vi "LFA_Close.vi"(8 "error in (no error)":errorcluster, 11 "LightField Automation in":refnum<class "LightField Automation.lvclass">) -> (0 "error out":errorcluster, 3 "LightField Automation out":refnum<class "LightField Automation.lvclass">)   [LabVIEW 2013, in "LightField Automation.lvclass"]
uses:
  LightField Automation.lvclass
  LightField Automation.lvclass/LightField Automation.ctl
  C:/Program Files/Princeton Instruments/LightField/PrincetonInstruments.LightField.AutomationV3.dll
  Program Files/Princeton Instruments/LightField/PrincetonInstruments.LightField.AutomationV3.dll
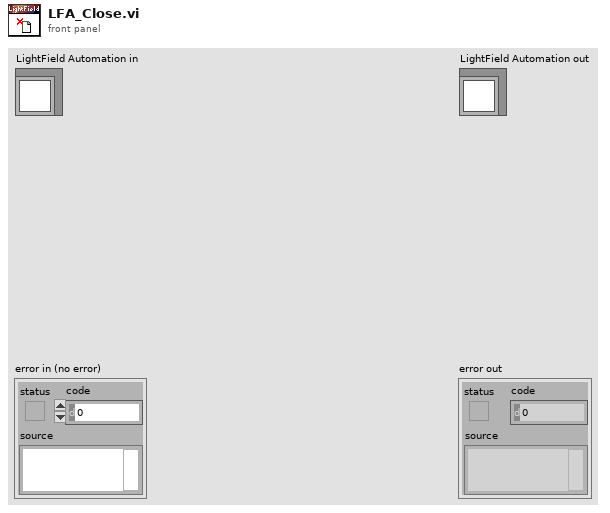
[diagram p1: front panel]
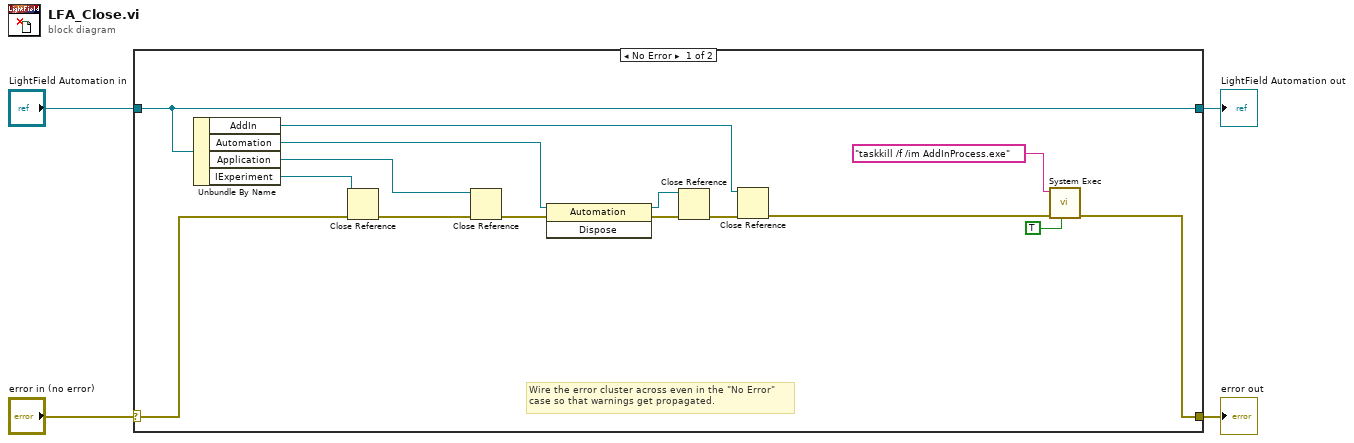
[diagram p0: block diagram]
diagram:
  n1 = case shown="No Error" "error in (no error)" {
    selector: "error in (no error)" -> [w15 w21]
    tunnel: [w6 w21] -> w3
    tunnel: [w19 w20] -> w1
    tunnel: "LightField Automation in" -> [w19 w20]
    frame No Error {
      # "Wire the error cluster across even in the \"No Error\"\ncase so that warnings get propagated."
      n2 = Unbundle By Name(w19) -> ("AddIn"=w10:refnum<k24>, "Automation"=w13:refnum<k24>, "Application"=w16:refnum<k24>, "IExperiment"=w17:refnum<k24>)
      n3 = Close Reference(reference=w17, error in (no error)=w15) -> (error out=w18:errorcluster)
      n4 = Close Reference(reference=w16, error in (no error)=w18) -> (error out=w11:errorcluster)
      n5 = invoke class="Automation" method="Dispose"(reference=w13, error in=w11) -> (reference out=w12:refnum<k24>, error out=w14:errorcluster)  [unwired: 1 in, 1 out]
      n6 = Close Reference(reference=w12, error in (no error)=w14) -> (error out=w9:errorcluster)
      n7 = Close Reference(reference=w10, error in (no error)=w9) -> (error out=w8:errorcluster)
      n8 = call <vilib>:"System Exec.vi"("run minimized? (F)"=TRUE, "error in (no error)"=w8, "command line"="taskkill /f /im AddInProcess.exe") -> ("error out"=w6:errorcluster)  [unwired: 5 in, 3 out]
    }
    frame Error {
    }
  }
  "error out" <- w3
  "LightField Automation out" <- w1
